vi "Do.vi"(8 "error in (no error)":errorcluster, 10 "Actor in":refnum<class "Actor.lvclass">, 11 "Message":refnum<class "Post Iteration Msg.lvclass">) -> (0 "error out":errorcluster, 2 "Actor out":refnum<class "Actor.lvclass">)   [LabVIEW 2021, in "Example Iterator NR Actor Explicit Iteration.lvlib" / "Post Iteration Msg.lvclass"]
doc: "(<B>Filename</B>: Actor Framework.lvlib:Reply Msg.lvclass:Do Core.vi)\n\nDefines what an actor does when it receives <B>Reply Message</B>. This method also defines the <B>Reply</B> that is returned to the actor that sent <B>Reply Message</B>.\n\nBy default, this method does nothing, and <B>Reply</B> is the ancestor Message class. A child class must override this method to define behavior and specify a child of the Message class to return in the <B>Reply</B> output."
uses:
  Post Iteration Msg.lvclass
  <vilib>/ActorFramework/Actor/Actor.lvclass
  Example Actor/Example Actor.lvclass
  C:/Program Files/National Instruments/LabVIEW 2021/vi.lib/ActorFramework/Actor/Actor.lvclass
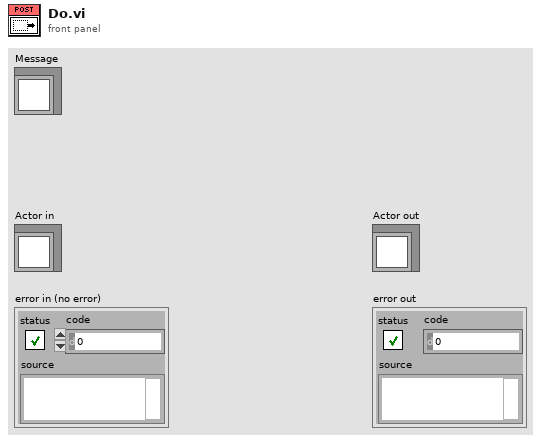
[diagram p1: front panel]
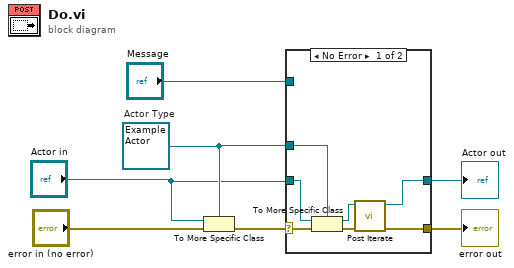
[diagram p0: block diagram]
diagram:
  w2 = refnum<class "Example Actor.lvclass"> refnum  # Actor Type
  n1 = To More Specific Class(target class=w2, reference="Actor in", error in="error in (no error)") -> (error out=w6:errorcluster)  [unwired: 1 out]
  n2 = case shown="No Error" w6 {
    selector: w6 -> [w14 w16]
    tunnel: [w10 w16] -> w3
    tunnel: [w9 w15] -> w4
    tunnel: "Actor in" -> [w13 w15]
    tunnel: w2 -> [w12 _]
    tunnel: "Message" -> [_ _]
    frame No Error {
      n3 = To More Specific Class ("Actor Cast")(target class=w12, reference=w13, error in=w14) -> (specific class reference=w8:refnum<class "Example Actor.lvclass">, error out=w11:errorcluster)
      n4 = call "Post Iterate.vi"("error in (no error)"=w11, "Example Actor in"=w8) -> ("error out"=w10:errorcluster, "Example Actor out"=w9:refnum<class "Example Actor.lvclass">)  [unwired: 8 in]
    }
    frame Error {
    }
  }
  "error out" <- w3
  "Actor out" <- w4
